vi "Write File Path.vi"(8 "error in (no error)":errorcluster, 10 "File Path":path, 11 "Worker in":refnum<class "Worker.lvclass">) -> (0 "error out":errorcluster, 3 "Worker out":refnum<class "Worker.lvclass">)   [LabVIEW 2016, in "Worker.lvclass"]
uses:
  Worker.lvclass
  Worker.lvclass/Worker.ctl
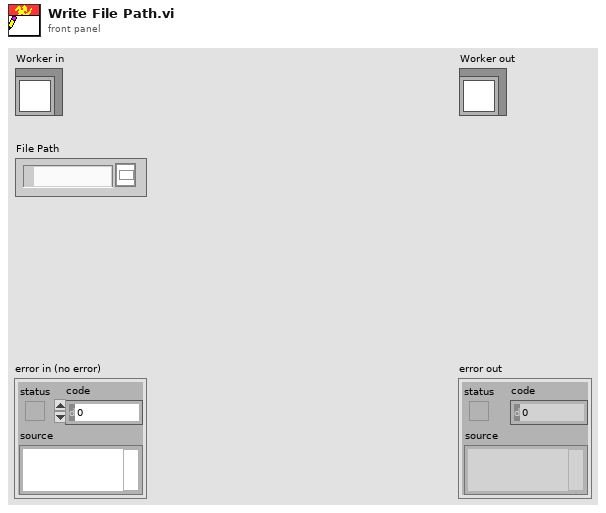
[diagram p1: front panel]
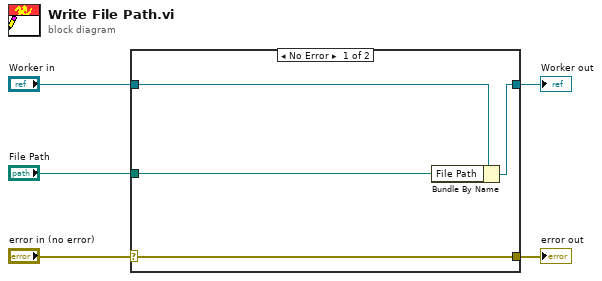
[diagram p0: block diagram]
diagram:
  n1 = case shown="No Error" "error in (no error)" {
    selector: "error in (no error)" -> [w9 w10]
    tunnel: [w9 w10] -> w4
    tunnel: [w7 w11] -> w2
    tunnel: "Worker in" -> [w8 w11]
    tunnel: "File Path" -> [w6 _]
    frame No Error {
      n2 = Bundle By Name(cluster=w8, "File Path"=w6) -> (w7:refnum<class "Worker.lvclass">)
    }
    frame Error {
    }
  }
  "error out" <- w4
  "Worker out" <- w2
